vi "APLUS 120V Evansville System.vi"(0 "Modbus Master in":refnum<class "Modbus Master.lvclass">, 3 "Power Input":T2 {"Voltage (V):Element 1 Avg" format="%.3g"; "Voltage (V):Element 2 Avg" format="%.3g"; "Max Watt Hours" format="%.3g"; "Power Factor:Element 2" format="%.3g"; "Power Factor:Element 1" format="%.3g"; "Apparent Power (VA):Element 2" format="%.3g"; "Apparent Power (VA):Element 1" format="%.3g"; "Frequency (Hz):Element 1" format="%.3g"; "Time:Element 1" format="%.3g"; "Voltage Crest Factor:Element 2" format="%.3g"; "Voltage Crest Factor:Element 1" format="%.3g"; "Voltage Harmonic (%):Element 2" format="%.3g"; "Voltage Harmonic (%):Element 1" format="%.3g"; "Current Crest Factor:Element 2" format="%.3g"; "Current Crest Factor:Element 1" format="%.3g"; "Voltage (V):Element 1" format="%.3g"; "Voltage (V):Element 2" format="%.3g"; "Watt Hours (Wh):Sigma" format="%.3f"; "Power (W):Sigma" format="%.3g"; "Current (A):Element 2" format="%.3g"; "Current (A):Element 1" format="%.3g"}, 11 "error in (no error)":errorcluster) -> (4 "Modbus Master out":refnum<class "Modbus Master.lvclass">, 6 "Holding Registers":u16[](array[numeric]), 8 "Power out":sgl, 10 "PowerData":T2 {"Voltage (V):Element 1 Avg" format="%.3g"; "Voltage (V):Element 2 Avg" format="%.3g"; "Max Watt Hours" format="%.3g"; "Power Factor:Element 2" format="%.3g"; "Power Factor:Element 1" format="%.3g"; "Apparent Power (VA):Element 2" format="%.3g"; "Apparent Power (VA):Element 1" format="%.3g"; "Frequency (Hz):Element 1" format="%.3g"; "Time:Element 1" format="%.3g"; "Voltage Crest Factor:Element 2" format="%.3g"; "Voltage Crest Factor:Element 1" format="%.3g"; "Voltage Harmonic (%):Element 2" format="%.3g"; "Voltage Harmonic (%):Element 1" format="%.3g"; "Current Crest Factor:Element 2" format="%.3g"; "Current Crest Factor:Element 1" format="%.3g"; "Voltage (V):Element 1" format="%.3g"; "Voltage (V):Element 2" format="%.3g"; "Watt Hours (Wh):Sigma" format="%.3f"; "Power (W):Sigma" format="%.3g"; "Current (A):Element 2" format="%.3g"; "Current (A):Element 1" format="%.3g"}, 15 "error out":errorcluster)   [LabVIEW 2016]
uses:
  <vilib>/NI/Modbus Library/API/Master/Modbus Master.lvclass
  C:/Program Files (x86)/National Instruments/LabVIEW 2016/vi.lib/NI/Modbus Library/API/Modbus API.lvclass
  Trunk/Utility/Type Definitions/UTILITY Power Data.ctl
  Type Definitions/APLUS Commands.ctl
panel:
  in  "Vthd":T1=235 items=["L1 Voltage (V) -14"=99, "L1 Voltage (V) -4U"=101, "L2 Voltage (V) -4U"=103, "L1 RMS Current (Amps) -14"=115, "L1 RMS Current (Amps) -4U"=117, "L2 RMS Current (Amps) -4U"=119, "Frequency (Hz) -All"=157, "Sys Power (Watts)-14"=133, "L1 Power (Watts)-4U"=135, "L2 Power (Watts)-4U"=137, "L1 Power Factor-14"=159, "L1 Power Factor-4U"=161, "L2 Power Factor-4U"=163, "L1 Apparent Power (VA)-14"=149, "L1 Apparent Power (VA)-4U"=151, "L2 Apparent Power (VA)-4U"=153, "Voltage Total Harmonic Distortion (%)-All"=235, "Active Energy Incoming-14"=1579, "Unit Factor-14"=1627, "Remainder Active Energy Incoming-14"=5999, "System Type"=2199]
  in  "Apparent Power":T1=151 items=["L1 Voltage (V) -14"=99, "L1 Voltage (V) -4U"=101, "L2 Voltage (V) -4U"=103, "L1 RMS Current (Amps) -14"=115, "L1 RMS Current (Amps) -4U"=117, "L2 RMS Current (Amps) -4U"=119, "Frequency (Hz) -All"=157, "Sys Power (Watts)-14"=133, "L1 Power (Watts)-4U"=135, "L2 Power (Watts)-4U"=137, "L1 Power Factor-14"=159, "L1 Power Factor-4U"=161, "L2 Power Factor-4U"=163, "L1 Apparent Power (VA)-14"=149, "L1 Apparent Power (VA)-4U"=151, "L2 Apparent Power (VA)-4U"=153, "Voltage Total Harmonic Distortion (%)-All"=235, "Active Energy Incoming-14"=1579, "Unit Factor-14"=1627, "Remainder Active Energy Incoming-14"=5999, "System Type"=2199]
  in  "Power Factor":T1=161 items=["L1 Voltage (V) -14"=99, "L1 Voltage (V) -4U"=101, "L2 Voltage (V) -4U"=103, "L1 RMS Current (Amps) -14"=115, "L1 RMS Current (Amps) -4U"=117, "L2 RMS Current (Amps) -4U"=119, "Frequency (Hz) -All"=157, "Sys Power (Watts)-14"=133, "L1 Power (Watts)-4U"=135, "L2 Power (Watts)-4U"=137, "L1 Power Factor-14"=159, "L1 Power Factor-4U"=161, "L2 Power Factor-4U"=163, "L1 Apparent Power (VA)-14"=149, "L1 Apparent Power (VA)-4U"=151, "L2 Apparent Power (VA)-4U"=153, "Voltage Total Harmonic Distortion (%)-All"=235, "Active Energy Incoming-14"=1579, "Unit Factor-14"=1627, "Remainder Active Energy Incoming-14"=5999, "System Type"=2199]
  in  "Power in":T1=135 items=["L1 Voltage (V) -14"=99, "L1 Voltage (V) -4U"=101, "L2 Voltage (V) -4U"=103, "L1 RMS Current (Amps) -14"=115, "L1 RMS Current (Amps) -4U"=117, "L2 RMS Current (Amps) -4U"=119, "Frequency (Hz) -All"=157, "Sys Power (Watts)-14"=133, "L1 Power (Watts)-4U"=135, "L2 Power (Watts)-4U"=137, "L1 Power Factor-14"=159, "L1 Power Factor-4U"=161, "L2 Power Factor-4U"=163, "L1 Apparent Power (VA)-14"=149, "L1 Apparent Power (VA)-4U"=151, "L2 Apparent Power (VA)-4U"=153, "Voltage Total Harmonic Distortion (%)-All"=235, "Active Energy Incoming-14"=1579, "Unit Factor-14"=1627, "Remainder Active Energy Incoming-14"=5999, "System Type"=2199]
  in  "Frequency":T1=157 items=["L1 Voltage (V) -14"=99, "L1 Voltage (V) -4U"=101, "L2 Voltage (V) -4U"=103, "L1 RMS Current (Amps) -14"=115, "L1 RMS Current (Amps) -4U"=117, "L2 RMS Current (Amps) -4U"=119, "Frequency (Hz) -All"=157, "Sys Power (Watts)-14"=133, "L1 Power (Watts)-4U"=135, "L2 Power (Watts)-4U"=137, "L1 Power Factor-14"=159, "L1 Power Factor-4U"=161, "L2 Power Factor-4U"=163, "L1 Apparent Power (VA)-14"=149, "L1 Apparent Power (VA)-4U"=151, "L2 Apparent Power (VA)-4U"=153, "Voltage Total Harmonic Distortion (%)-All"=235, "Active Energy Incoming-14"=1579, "Unit Factor-14"=1627, "Remainder Active Energy Incoming-14"=5999, "System Type"=2199]
  in  "Current":T1=117 items=["L1 Voltage (V) -14"=99, "L1 Voltage (V) -4U"=101, "L2 Voltage (V) -4U"=103, "L1 RMS Current (Amps) -14"=115, "L1 RMS Current (Amps) -4U"=117, "L2 RMS Current (Amps) -4U"=119, "Frequency (Hz) -All"=157, "Sys Power (Watts)-14"=133, "L1 Power (Watts)-4U"=135, "L2 Power (Watts)-4U"=137, "L1 Power Factor-14"=159, "L1 Power Factor-4U"=161, "L2 Power Factor-4U"=163, "L1 Apparent Power (VA)-14"=149, "L1 Apparent Power (VA)-4U"=151, "L2 Apparent Power (VA)-4U"=153, "Voltage Total Harmonic Distortion (%)-All"=235, "Active Energy Incoming-14"=1579, "Unit Factor-14"=1627, "Remainder Active Energy Incoming-14"=5999, "System Type"=2199]
  in  "Voltage (L1-N)":T1=101 items=["L1 Voltage (V) -14"=99, "L1 Voltage (V) -4U"=101, "L2 Voltage (V) -4U"=103, "L1 RMS Current (Amps) -14"=115, "L1 RMS Current (Amps) -4U"=117, "L2 RMS Current (Amps) -4U"=119, "Frequency (Hz) -All"=157, "Sys Power (Watts)-14"=133, "L1 Power (Watts)-4U"=135, "L2 Power (Watts)-4U"=137, "L1 Power Factor-14"=159, "L1 Power Factor-4U"=161, "L2 Power Factor-4U"=163, "L1 Apparent Power (VA)-14"=149, "L1 Apparent Power (VA)-4U"=151, "L2 Apparent Power (VA)-4U"=153, "Voltage Total Harmonic Distortion (%)-All"=235, "Active Energy Incoming-14"=1579, "Unit Factor-14"=1627, "Remainder Active Energy Incoming-14"=5999, "System Type"=2199]
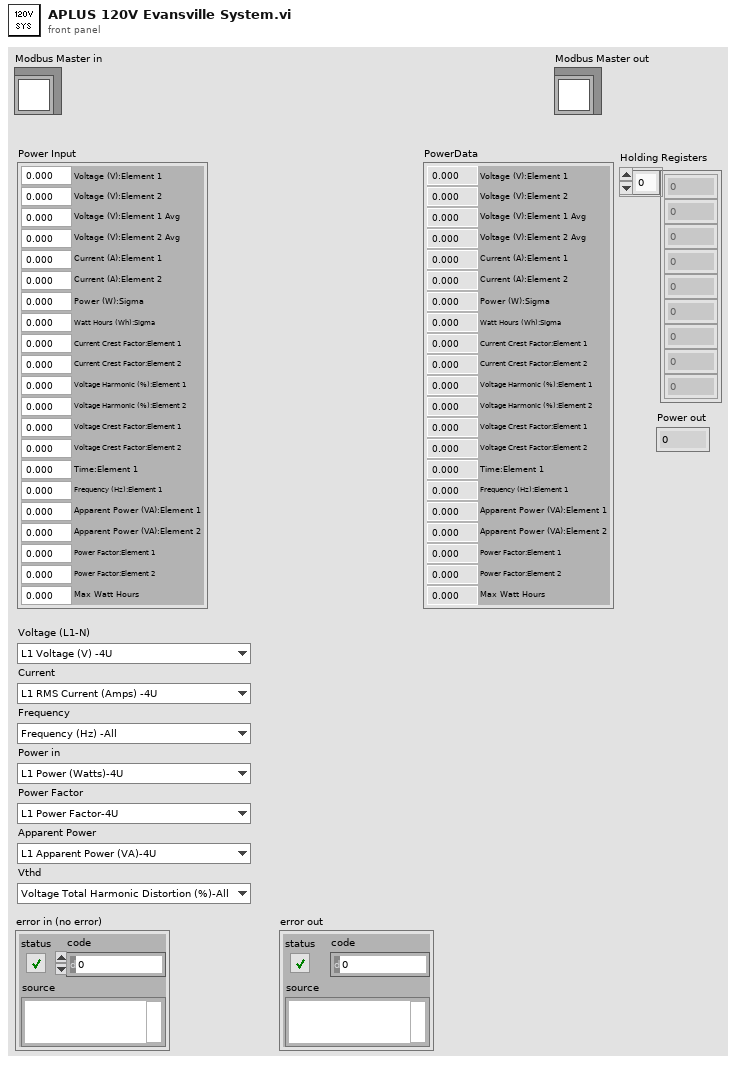
[diagram p1: front panel]
types:
  T1 = typedef "APLUS Commands.ctl" = u16
  T2 = typedef "UTILITY Power Data.ctl" = cluster{"Current (A):Element 1":dbl, "Current (A):Element 2":dbl, "Power (W):Sigma":dbl, "Watt Hours (Wh):Sigma":dbl, "Voltage (V):Element 2":dbl, "Voltage (V):Element 1":dbl, "Current Crest Factor:Element 1":dbl, "Current Crest Factor:Element 2":dbl, "Voltage Harmonic (%):Element 1":dbl, "Voltage Harmonic (%):Element 2":dbl, "Voltage Crest Factor:Element 1":dbl, "Voltage Crest Factor:Element 2":dbl, "Time:Element 1":dbl, "Frequency (Hz):Element 1":dbl, "Apparent Power (VA):Element 1":dbl, "Apparent Power (VA):Element 2":dbl, "Power Factor:Element 1":dbl, "Power Factor:Element 2":dbl, "Max Watt Hours":dbl, "Voltage (V):Element 2 Avg":dbl, "Voltage (V):Element 1 Avg":dbl}
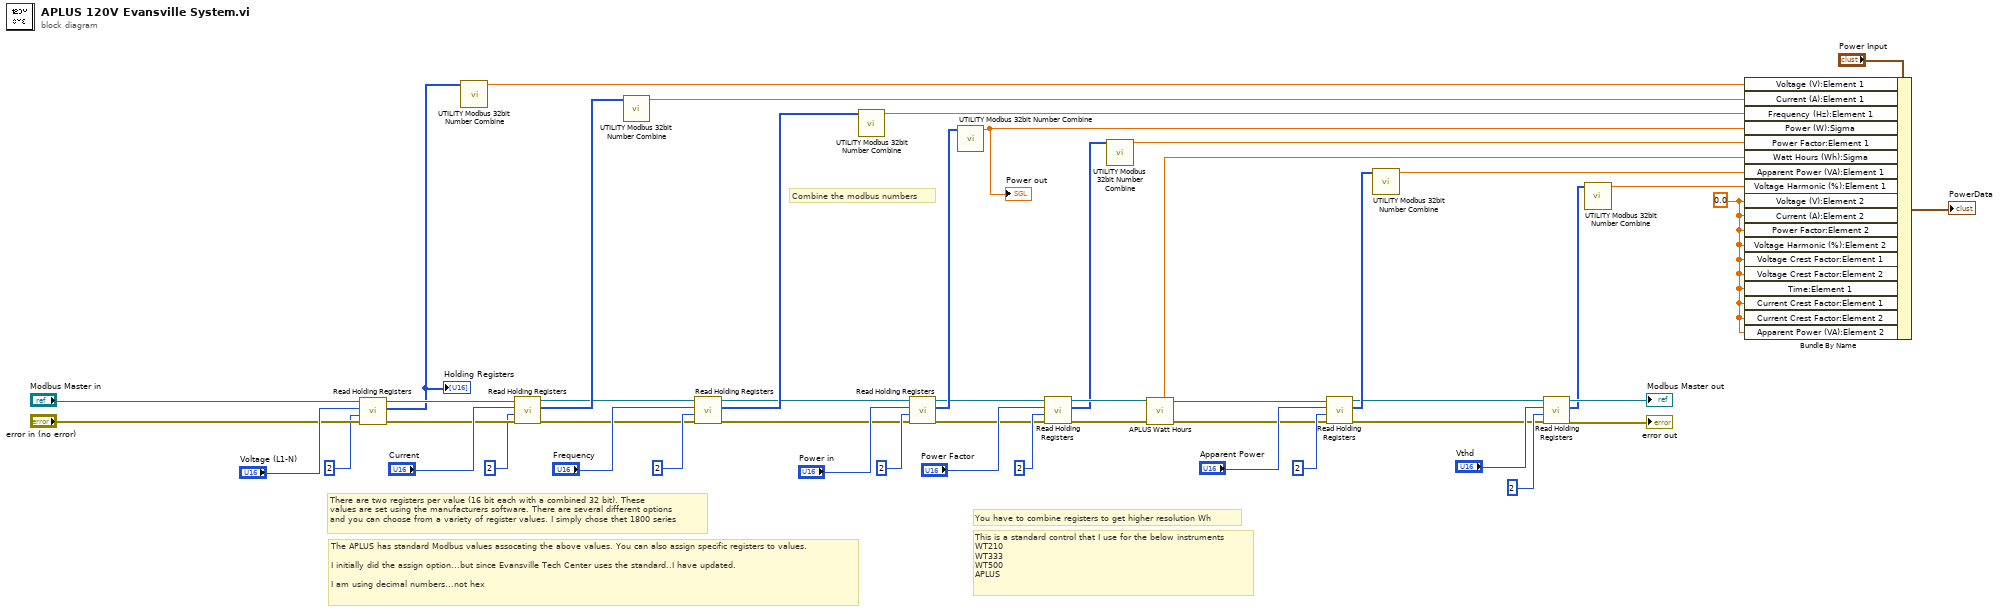
[diagram p0: block diagram]
diagram:
  w49 = 0.0 ("Urms:Element 2")
  # "The APLUS has standard Modbus values assocating the above values. You can also assign specific registers to values.\n\nI initially did the assign option...but since Evansville Tech Center uses the standard..I have updated.\n\nI am using decimal numbers...not hex"
  # "You have to combine registers to get higher resolution Wh"
  # "This is a standard control that I use for the below instruments\nWT210\nWT333\nWT500\nAPLUS"
  # "Combine the modbus numbers"
  # "There are two registers per value (16 bit each with a combined 32 bit). These \nvalues are set using the manufacturers software. There are several different options\nand you can choose from a variety of register values. I simply chose thet 1800 series"
  n1 = call-dynamic "Read Holding Registers.vi"("error in"="error in (no error)", "number of inputs"=u16 2 ("Quantity"), "starting address"="Voltage (L1-N)", "Modbus master in"="Modbus Master in") -> ("error out"=w21:errorcluster, "register values"=w18:u16[], "Modbus master out"=w19:refnum<class "Modbus Master.lvclass">)  [unwired: 5 in]
  "Holding Registers" <- w18
  n2 = call "UTILITY Modbus 32bit Number Combine.vi"("Holding Registers"=w18) -> ("Data"=w41:sgl)  [unwired: 9 in, 1 out]
  n3 = call-dynamic "Read Holding Registers.vi"("error in"=w21, "number of inputs"=u16 2 ("Quantity"), "starting address"="Current", "Modbus master in"=w19) -> ("error out"=w9:errorcluster, "register values"=w28:u16[], "Modbus master out"=w5:refnum<class "Modbus Master.lvclass">)  [unwired: 5 in]
  n4 = call "UTILITY Modbus 32bit Number Combine.vi"("Holding Registers"=w28) -> ("Data"=w42:sgl)  [unwired: 9 in, 1 out]
  n5 = call-dynamic "Read Holding Registers.vi"("error in"=w9, "number of inputs"=u16 2 ("Quantity"), "starting address"="Frequency", "Modbus master in"=w5) -> ("error out"=w8:errorcluster, "register values"=w7:u16[], "Modbus master out"=w4:refnum<class "Modbus Master.lvclass">)  [unwired: 5 in]
  n6 = call "UTILITY Modbus 32bit Number Combine.vi"("Holding Registers"=w7) -> ("Data"=w43:sgl)  [unwired: 9 in, 1 out]
  n7 = call-dynamic "Read Holding Registers.vi"("error in"=w8, "number of inputs"=u16 2 ("Quantity"), "starting address"="Power in", "Modbus master in"=w4) -> ("error out"=w3:errorcluster, "register values"=w6:u16[], "Modbus master out"=w1:refnum<class "Modbus Master.lvclass">)  [unwired: 5 in]
  n8 = call "UTILITY Modbus 32bit Number Combine.vi"("Holding Registers"=w6) -> ("Data"=w44:sgl)  [unwired: 9 in, 1 out]
  "Power out" <- w44
  n9 = call-dynamic "Read Holding Registers.vi"("error in"=w3, "number of inputs"=u16 2 ("Quantity"), "starting address"="Power Factor", "Modbus master in"=w1) -> ("error out"=w10:errorcluster, "register values"=w2:u16[], "Modbus master out"=w11:refnum<class "Modbus Master.lvclass">)  [unwired: 5 in]
  n10 = call "UTILITY Modbus 32bit Number Combine.vi"("Holding Registers"=w2) -> ("Data"=w45:sgl)  [unwired: 9 in, 1 out]
  n11 = call "APLUS Watt Hours.vi"("error in (no error)"=w10, "Modbus instance in"=w11) -> ("error out"=w14:errorcluster, "Modbus instance out"=w16:refnum<class "Modbus Master.lvclass">, "Watt Hours"=w46:dbl)  [unwired: 7 in]
  n12 = call-dynamic "Read Holding Registers.vi"("error in"=w14, "number of inputs"=u16 2 ("Quantity"), "starting address"="Apparent Power", "Modbus master in"=w16) -> ("error out"=w15:errorcluster, "register values"=w13:u16[], "Modbus master out"=w12:refnum<class "Modbus Master.lvclass">)  [unwired: 5 in]
  n13 = call "UTILITY Modbus 32bit Number Combine.vi"("Holding Registers"=w13) -> ("Data"=w47:sgl)  [unwired: 9 in, 1 out]
  n14 = call-dynamic "Read Holding Registers.vi"("error in"=w15, "number of inputs"=u16 2 ("Quantity"), "starting address"="Vthd", "Modbus master in"=w12) -> ("error out"=→"error out":errorcluster, "register values"=w27:u16[], "Modbus master out"=→"Modbus Master out":refnum<class "Modbus Master.lvclass">)  [unwired: 5 in]
  n15 = call "UTILITY Modbus 32bit Number Combine.vi"("Holding Registers"=w27) -> ("Data"=w48:sgl)  [unwired: 9 in, 1 out]
  n16 = Bundle By Name(cluster="Power Input", "Voltage (V):Element 1"=w41, "Current (A):Element 1"=w42, "Frequency (Hz):Element 1"=w43, "Power (W):Sigma"=w44, "Power Factor:Element 1"=w45, "Watt Hours (Wh):Sigma"=w46, "Apparent Power (VA):Element 1"=w47, "Voltage Harmonic (%):Element 1"=w48, "Voltage (V):Element 2"=w49, "Current (A):Element 2"=w49, "Power Factor:Element 2"=w49, "Voltage Harmonic (%):Element 2"=w49, "Voltage Crest Factor:Element 1"=w49, "Voltage Crest Factor:Element 2"=w49, "Time:Element 1"=w49, "Current Crest Factor:Element 1"=w49, "Current Crest Factor:Element 2"=w49, "Apparent Power (VA):Element 2"=w49) -> (→"PowerData":T2)
